vi "Demo_Dynamic.vi"() -> ()   [LabVIEW 2012]
uses:
  WaveGraphX.xctl
panel:
  in  "停止按钮":bool
  out "WaveGraphX":dbl[][](xcontrol)
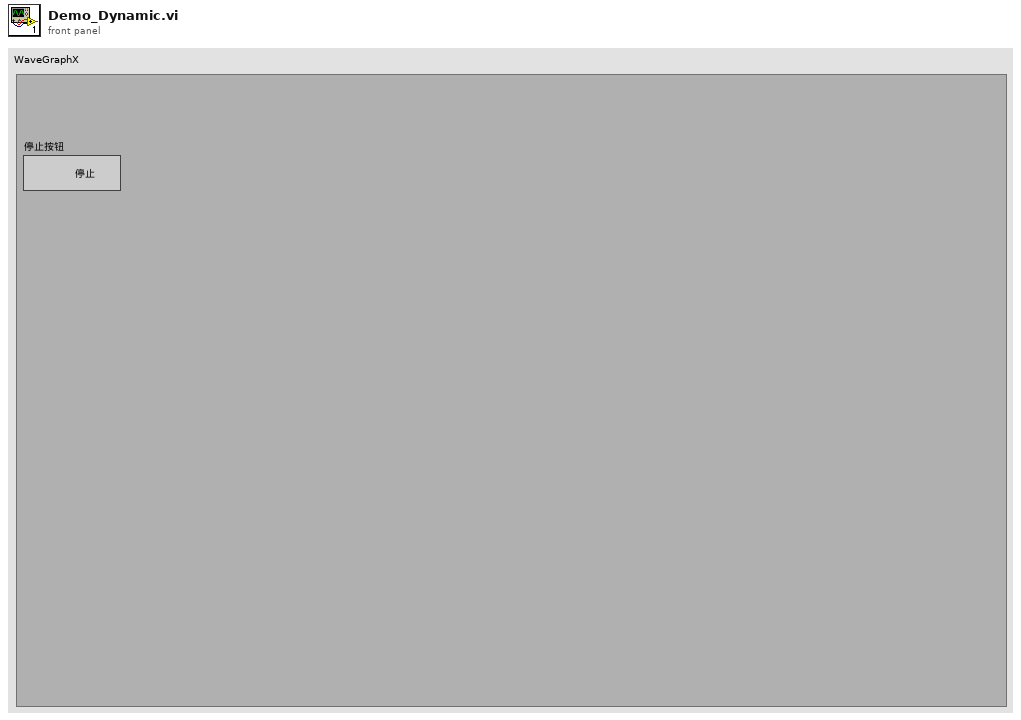
[diagram p1: front panel]
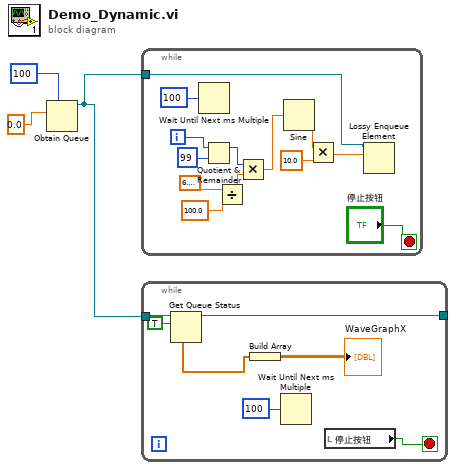
[diagram p0: block diagram]
diagram:
  n1 = Obtain Queue(max queue size (-1, unlimited)=100 ("队列最大值（-1，无限）"), element data type=0.0) -> (queue out=w1:refnum<queue>)  [unwired: 3 in, 2 out]
  n2 = while {
    tunnel: w1 -> [w9]
    i -> [w16]
    stop <- "停止按钮" stop-if-true
    n3 = Wait Until Next ms Multiple(millisecond multiple=u32 100 ("毫秒倍数")) -> ()  [unwired: 1 out]
    n4 = Quotient & Remainder(x=w16, y=99) -> (x-y*floor(x/y)=w6:i32)  [unwired: 1 out]
    n5 = Divide(x=6.283185307179586, y=100.0) -> (x/y=w5:dbl)
    n6 = Multiply(x=w6, y=w5) -> (x*y=w4:dbl)
    n7 = Sine(x=w4) -> (sin(x)=w12:dbl)
    n8 = Multiply(x=w12, y=10.0) -> (x*y=w8:dbl)
    n9 = Lossy Enqueue Element(queue=w9, element=w8) -> ()  [unwired: 1 in, 4 out]
  }
  n10 = while {
    tunnel: w1 -> [w22]
    tunnel: [w20] -> _
    stop <- w23 stop-if-true
    n11 = Get Queue Status(queue=w22, return elements? (F)=TRUE ("返回元素？(F)")) -> (queue out=w20:refnum<queue>, elements=w18:dbl[])  [unwired: 1 in, 6 out]
    n12 = Build Array(w18) -> (→"WaveGraphX":dbl[][])
    n13 = Wait Until Next ms Multiple(millisecond multiple=u32 100 ("毫秒倍数")) -> ()  [unwired: 1 out]
    n14 = local read "停止按钮"() -> (w23:bool)
  }
